vi "capex gui.vi"() -> ()   [LabVIEW 2013]
panel:
  in  "On quit":bool
  out "Heartbeat":bool
  in  "Tab Control":T1(tab)
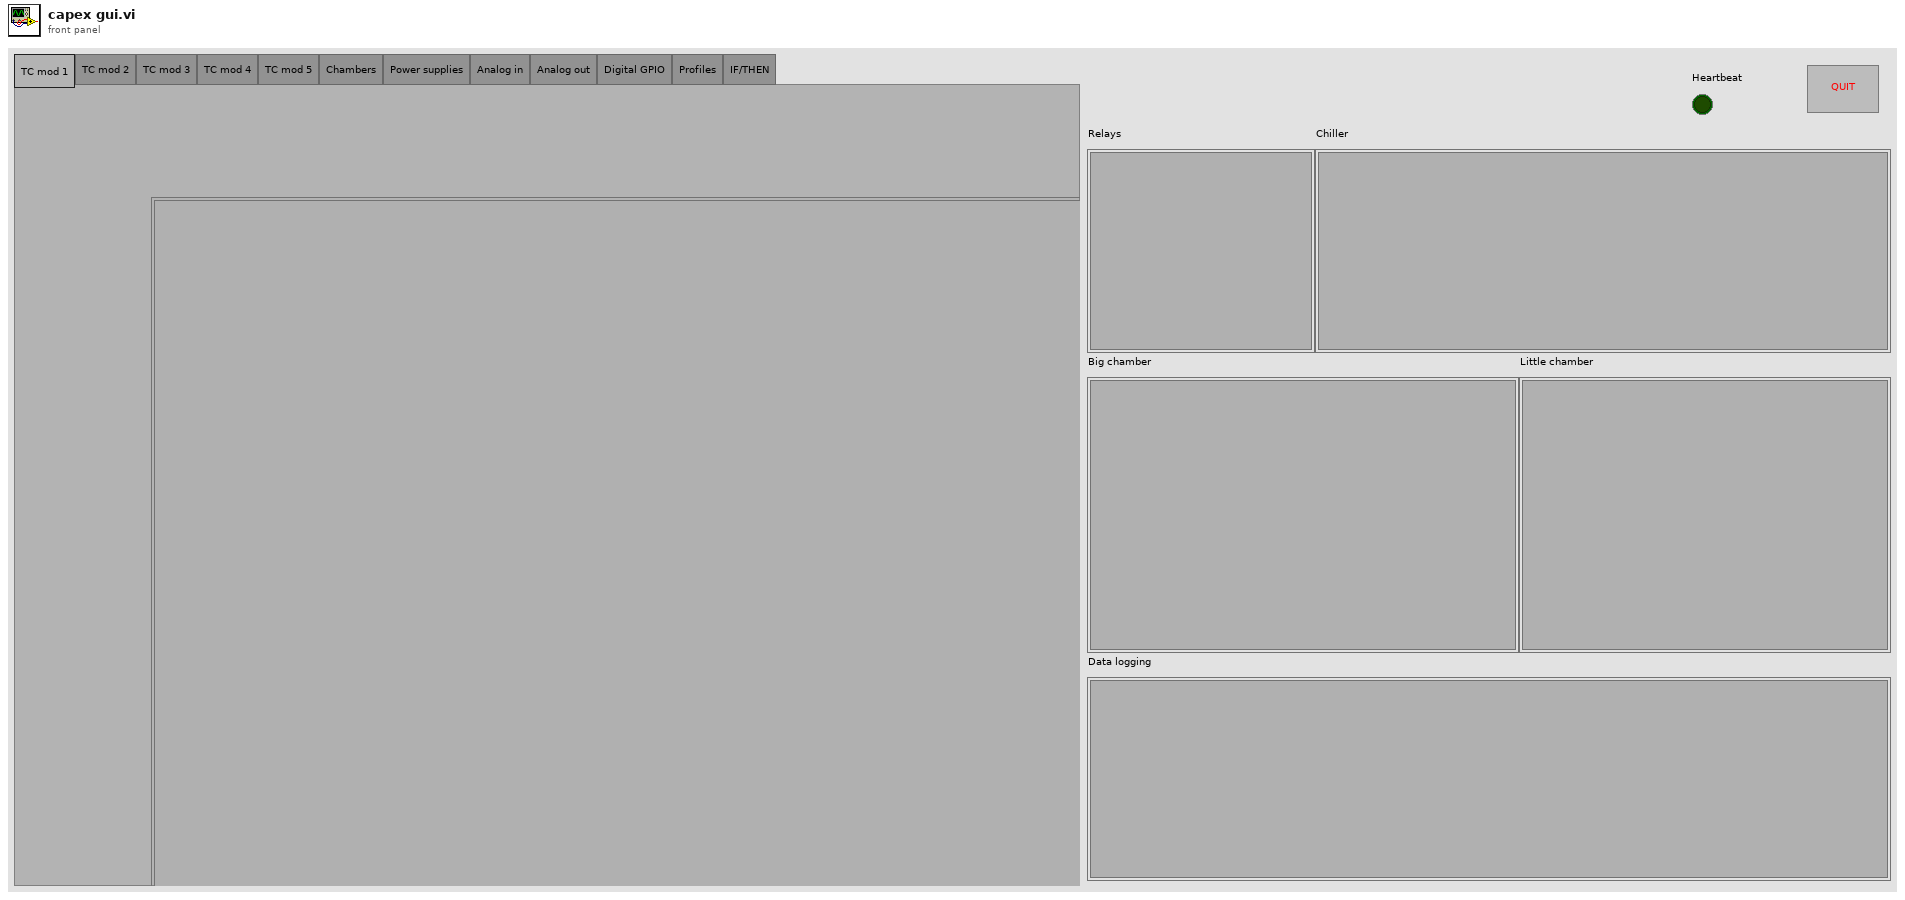
[diagram p1: front panel]
types:
  T1 = enum32{"TC mod 1", "TC mod 2", "TC mod 3", "TC mod 4", "TC mod 5", "Chambers", "Power supplies", "Analog in", "Analog out", "Digital GPIO", "Profiles", "IF/THEN"}
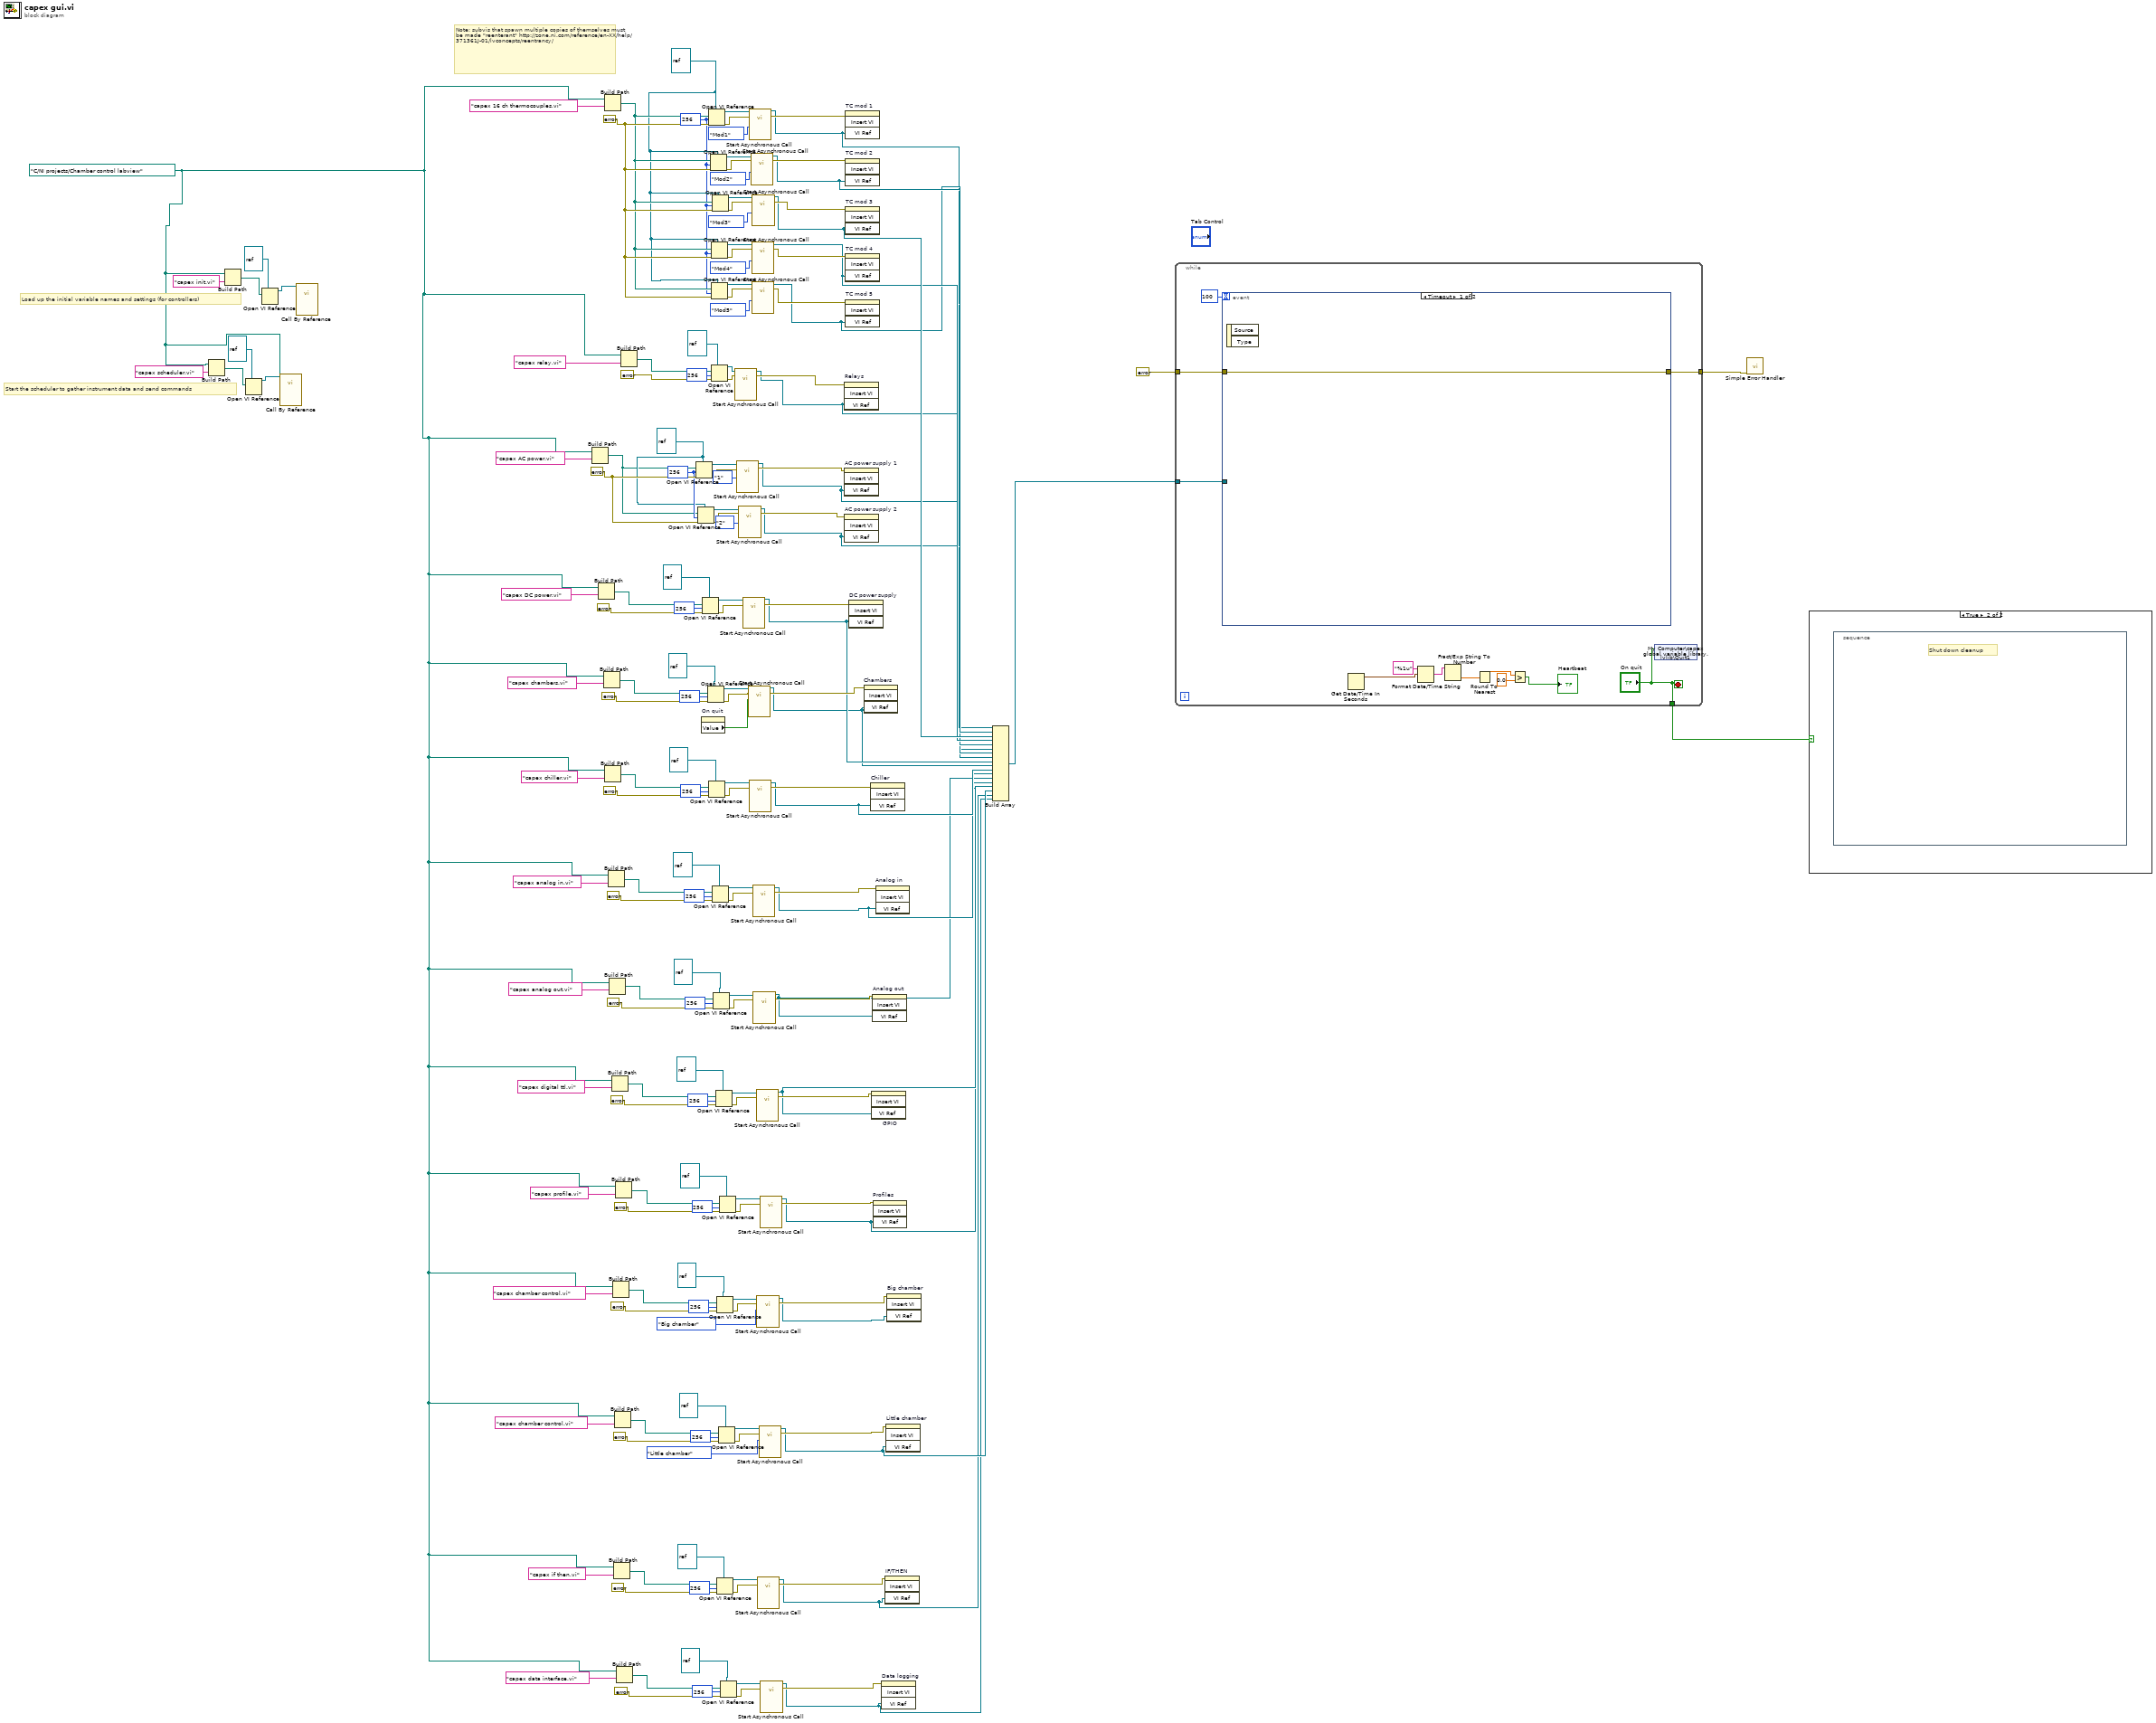
[diagram p0: block diagram]
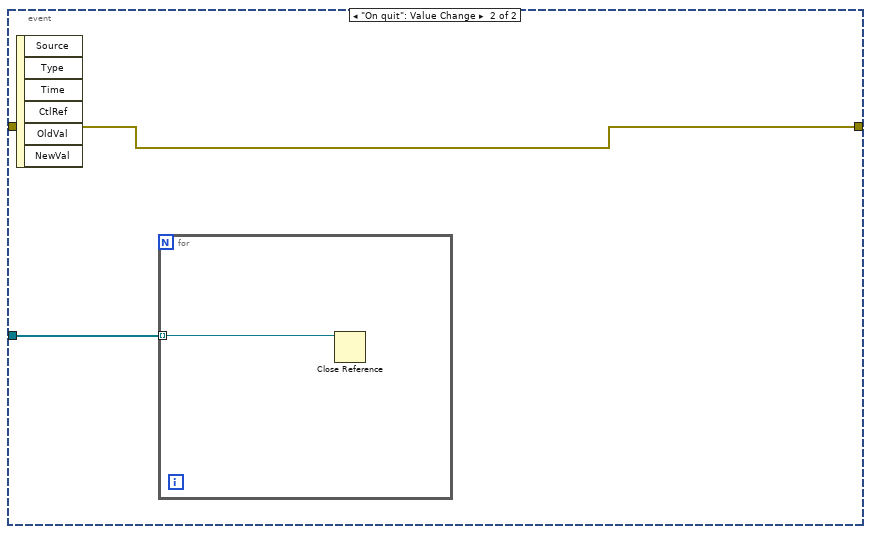
[diagram p3: hidden frame]
diagram:
  w138 = 256 ("options")
  w135 = refnum<vi> refnum ("type specifier VI Refnum (for type only)")
  w141 = errorcluster {"status"=FALSE, "code"=0, "source"=""} ("error out")
  w147 = 256 ("options")
  w148 = refnum<vi> refnum ("type specifier VI Refnum (for type only)")
  w162 = errorcluster {"status"=FALSE, "code"=0, "source"=""} ("error out")
  w11 = path "C:/NI projects/Chamber control labview"
  # "Start the scheduler to gather instrument data and send commands"
  # "Load up the initial variable names and settings (for controllers)"
  # "Note: subvis that spawn multiple copies of themselves must be made \"reenterant\" http://zone.ni.com/reference/en-XX/help/371361J-01/lvconcepts/reentrancy/"
  n1 = Build Path(base path=w11, name or relative path="capex scheduler.vi") -> (appended path=w5:path)
  n2 = Build Path(base path=w11, name or relative path="capex init.vi") -> (appended path=w9:path)
  n3 = Open VI Reference(type specifier VI Refnum (for type only)=refnum<vi> refnum, vi path=w5) -> (vi reference=w3:refnum<vi>)  [unwired: 4 in, 1 out]
  n4 = Open VI Reference(type specifier VI Refnum (for type only)=refnum<vi> refnum, vi path=w9) -> (vi reference=w7:refnum<vi>)  [unwired: 4 in, 1 out]
  n5 = call-by-ref "?"(reference=w3, "Path"=w11) -> ()  [unwired: 12 in, 2 out]
  n6 = call-by-ref "?"(reference=w7) -> ()  [unwired: 2 in, 11 out]
  n7 = Build Path(base path=w11, name or relative path="capex AC power.vi") -> (appended path=w134:path)
  n8 = Build Path(base path=w11, name or relative path="capex DC power.vi") -> (appended path=w119:path)
  n9 = Build Path(base path=w11, name or relative path="capex chambers.vi") -> (appended path=w111:path)
  n10 = Build Path(base path=w11, name or relative path="capex 16 ch thermocouples.vi") -> (appended path=w149:path)
  n11 = Build Path(base path=w11, name or relative path="capex chiller.vi") -> (appended path=w104:path)
  n12 = Build Path(base path=w11, name or relative path="capex analog in.vi") -> (appended path=w97:path)
  n13 = Build Path(base path=w11, name or relative path="capex analog out.vi") -> (appended path=w90:path)
  n14 = Build Path(base path=w11, name or relative path="capex digital ttl.vi") -> (appended path=w83:path)
  n15 = Build Path(base path=w11, name or relative path="capex chamber control.vi") -> (appended path=w44:path)
  n16 = Build Path(base path=w11, name or relative path="capex if then.vi") -> (appended path=w63:path)
  n17 = Build Path(base path=w11, name or relative path="capex chamber control.vi") -> (appended path=w37:path)
  n18 = Build Path(base path=w11, name or relative path="capex profile.vi") -> (appended path=w76:path)
  n19 = Build Path(base path=w11, name or relative path="capex data interface.vi") -> (appended path=w56:path)
  n20 = Build Path(base path=w11, name or relative path="capex relay.vi") -> (appended path=w168:path)
  n21 = Open VI Reference(type specifier VI Refnum (for type only)=w135, vi path=w134, options=w138, error in (no error)=w141) -> (vi reference=w143:refnum<vi>, error out=w142:errorcluster)  [unwired: 2 in]
  n22 = Open VI Reference(type specifier VI Refnum (for type only)=w135, vi path=w134, options=w138, error in (no error)=w141) -> (vi reference=w140:refnum<vi>, error out=w139:errorcluster)  [unwired: 2 in]
  n23 = property on="On quit" class="Bool (strict)"() -> ("Value"=w51:bool)  [unwired: 2 in, 2 out]
  n24 = Open VI Reference(type specifier VI Refnum (for type only)=refnum<vi> refnum, vi path=w119, options=256, error in (no error)=errorcluster {"status"=FALSE, "code"=0, "source"=""} ("error out")) -> (vi reference=w124:refnum<vi>, error out=w123:errorcluster)  [unwired: 2 in]
  n25 = Open VI Reference(type specifier VI Refnum (for type only)=refnum<vi> refnum, vi path=w111, options=256, error in (no error)=errorcluster {"status"=FALSE, "code"=0, "source"=""} ("error out")) -> (vi reference=w116:refnum<vi>, error out=w115:errorcluster)  [unwired: 2 in]
  n26 = Open VI Reference(type specifier VI Refnum (for type only)=w148, vi path=w149, options=w147, error in (no error)=w162) -> (vi reference=w165:refnum<vi>, error out=w164:errorcluster)  [unwired: 2 in]
  n27 = Open VI Reference(type specifier VI Refnum (for type only)=refnum<vi> refnum, vi path=w104, options=256, error in (no error)=errorcluster {"status"=FALSE, "code"=0, "source"=""} ("error out")) -> (vi reference=w109:refnum<vi>, error out=w108:errorcluster)  [unwired: 2 in]
  n28 = Open VI Reference(type specifier VI Refnum (for type only)=w148, vi path=w149, options=w147, error in (no error)=w162) -> (vi reference=w161:refnum<vi>, error out=w154:errorcluster)  [unwired: 2 in]
  n29 = Open VI Reference(type specifier VI Refnum (for type only)=w148, vi path=w149, options=w147, error in (no error)=w162) -> (vi reference=w159:refnum<vi>, error out=w156:errorcluster)  [unwired: 2 in]
  n30 = Open VI Reference(type specifier VI Refnum (for type only)=w148, vi path=w149, options=w147, error in (no error)=w162) -> (vi reference=w158:refnum<vi>, error out=w157:errorcluster)  [unwired: 2 in]
  n31 = Open VI Reference(type specifier VI Refnum (for type only)=refnum<vi> refnum, vi path=w168, options=256, error in (no error)=errorcluster {"status"=FALSE, "code"=0, "source"=""} ("error out")) -> (vi reference=w14:refnum<vi>, error out=w15:errorcluster)  [unwired: 2 in]
  n32 = Open VI Reference(type specifier VI Refnum (for type only)=w148, vi path=w149, options=w147, error in (no error)=w162) -> (vi reference=w160:refnum<vi>, error out=w155:errorcluster)  [unwired: 2 in]
  n33 = Open VI Reference(type specifier VI Refnum (for type only)=refnum<vi> refnum, vi path=w97, options=256, error in (no error)=errorcluster {"status"=FALSE, "code"=0, "source"=""} ("error out")) -> (vi reference=w102:refnum<vi>, error out=w101:errorcluster)  [unwired: 2 in]
  n34 = Open VI Reference(type specifier VI Refnum (for type only)=refnum<vi> refnum, vi path=w90, options=256, error in (no error)=errorcluster {"status"=FALSE, "code"=0, "source"=""} ("error out")) -> (vi reference=w95:refnum<vi>, error out=w94:errorcluster)  [unwired: 2 in]
  n35 = Open VI Reference(type specifier VI Refnum (for type only)=refnum<vi> refnum, vi path=w83, options=256, error in (no error)=errorcluster {"status"=FALSE, "code"=0, "source"=""} ("error out")) -> (vi reference=w88:refnum<vi>, error out=w87:errorcluster)  [unwired: 2 in]
  n36 = Open VI Reference(type specifier VI Refnum (for type only)=refnum<vi> refnum, vi path=w44, options=256, error in (no error)=errorcluster {"status"=FALSE, "code"=0, "source"=""} ("error out")) -> (vi reference=w49:refnum<vi>, error out=w48:errorcluster)  [unwired: 2 in]
  n37 = Open VI Reference(type specifier VI Refnum (for type only)=refnum<vi> refnum, vi path=w63, options=256, error in (no error)=errorcluster {"status"=FALSE, "code"=0, "source"=""} ("error out")) -> (vi reference=w68:refnum<vi>, error out=w67:errorcluster)  [unwired: 2 in]
  n38 = Open VI Reference(type specifier VI Refnum (for type only)=refnum<vi> refnum, vi path=w37, options=256, error in (no error)=errorcluster {"status"=FALSE, "code"=0, "source"=""} ("error out")) -> (vi reference=w42:refnum<vi>, error out=w41:errorcluster)  [unwired: 2 in]
  n39 = Open VI Reference(type specifier VI Refnum (for type only)=refnum<vi> refnum, vi path=w76, options=256, error in (no error)=errorcluster {"status"=FALSE, "code"=0, "source"=""} ("error out")) -> (vi reference=w81:refnum<vi>, error out=w80:errorcluster)  [unwired: 2 in]
  n40 = Open VI Reference(type specifier VI Refnum (for type only)=refnum<vi> refnum, vi path=w56, options=256, error in (no error)=errorcluster {"status"=FALSE, "code"=0, "source"=""} ("error out")) -> (vi reference=w61:refnum<vi>, error out=w60:errorcluster)  [unwired: 2 in]
  n41 = call-by-ref "Start Asynchronous Call"(reference=w14, error in=w15) -> (reference out=w12:refnum<vi>, error out=w13:errorcluster)  [unwired: 4 in]
  n42 = call-by-ref "Start Asynchronous Call"(reference=w143, error in=w142, "Enum"=enum16{"2", "1"}."1") -> (reference out=w128:refnum<vi>, error out=w137:errorcluster)  [unwired: 3 in]
  n43 = call-by-ref "Start Asynchronous Call"(reference=w140, error in=w139, "Enum"=enum16{"2", "1"}."2") -> (reference out=w127:refnum<vi>, error out=w136:errorcluster)  [unwired: 3 in]
  n44 = call-by-ref "Start Asynchronous Call"(reference=w124, error in=w123) -> (reference out=w31:refnum<vi>, error out=w118:errorcluster)  [unwired: 4 in]
  n45 = call-by-ref "Start Asynchronous Call"(reference=w116, error in=w115, "stop"=w51) -> (reference out=w30:refnum<vi>, error out=w75:errorcluster)  [unwired: 11 in]
  n46 = call-by-ref "Start Asynchronous Call"(reference=w165, error in=w164, "Enum"=enum16{"Mod1", "Mod2", "Mod3", "Mod4", "Mod5"}."Mod1") -> (reference out=w53:refnum<vi>, error out=w163:errorcluster)  [unwired: 11 in]
  n47 = call-by-ref "Start Asynchronous Call"(reference=w109, error in=w108) -> (reference out=w29:refnum<vi>, error out=w74:errorcluster)  [unwired: 1 in]
  n48 = call-by-ref "Start Asynchronous Call"(reference=w161, error in=w154, "Enum"=enum16{"Mod1", "Mod2", "Mod3", "Mod4", "Mod5"}."Mod2") -> (reference out=w132:refnum<vi>, error out=w153:errorcluster)  [unwired: 11 in]
  n49 = call-by-ref "Start Asynchronous Call"(reference=w159, error in=w156, "Enum"=enum16{"Mod1", "Mod2", "Mod3", "Mod4", "Mod5"}."Mod4") -> (reference out=w130:refnum<vi>, error out=w151:errorcluster)  [unwired: 11 in]
  n50 = call-by-ref "Start Asynchronous Call"(reference=w158, error in=w157, "Enum"=enum16{"Mod1", "Mod2", "Mod3", "Mod4", "Mod5"}."Mod5") -> (reference out=w129:refnum<vi>, error out=w150:errorcluster)  [unwired: 11 in]
  n51 = call-by-ref "Start Asynchronous Call"(reference=w160, error in=w155, "Enum"=enum16{"Mod1", "Mod2", "Mod3", "Mod4", "Mod5"}."Mod3") -> (reference out=w131:refnum<vi>, error out=w152:errorcluster)  [unwired: 11 in]
  n52 = call-by-ref "Start Asynchronous Call"(reference=w102, error in=w101) -> (reference out=w28:refnum<vi>, error out=w73:errorcluster)  [unwired: 1 in]
  n53 = call-by-ref "Start Asynchronous Call"(reference=w95, error in=w94) -> (reference out=w27:refnum<vi>, error out=w72:errorcluster)  [unwired: 4 in]
  n54 = call-by-ref "Start Asynchronous Call"(reference=w88, error in=w87) -> (reference out=w26:refnum<vi>, error out=w71:errorcluster)  [unwired: 1 in]
  n55 = call-by-ref "Start Asynchronous Call"(reference=w49, error in=w48, "Which chamber"=enum16{"Little chamber", "Big chamber"}."Big chamber") -> (reference out=w35:refnum<vi>, error out=w36:errorcluster)  [unwired: 11 in]
  n56 = call-by-ref "Start Asynchronous Call"(reference=w68, error in=w67) -> (reference out=w23:refnum<vi>, error out=w55:errorcluster)  [unwired: 12 in]
  n57 = call-by-ref "Start Asynchronous Call"(reference=w42, error in=w41, "Which chamber"=enum16{"Little chamber", "Big chamber"}."Little chamber") -> (reference out=w24:refnum<vi>, error out=w34:errorcluster)  [unwired: 11 in]
  n58 = call-by-ref "Start Asynchronous Call"(reference=w81, error in=w80) -> (reference out=w25:refnum<vi>, error out=w70:errorcluster)  [unwired: 12 in]
  n59 = call-by-ref "Start Asynchronous Call"(reference=w61, error in=w60) -> (reference out=w22:refnum<vi>, error out=w54:errorcluster)  [unwired: 12 in]
  n60 = invoke on="Relays" class="SubPanel" method="Insert VI"(error in=w13, "VI Ref"=w12) -> ()  [unwired: 2 in, 4 out]
  n61 = invoke on="AC power supply 1" class="SubPnl" method="Insert VI"(error in=w137, "VI Ref"=w128) -> ()  [unwired: 2 in, 4 out]
  n62 = invoke on="AC power supply 2" class="SubPanel" method="Insert VI"(error in=w136, "VI Ref"=w127) -> ()  [unwired: 2 in, 4 out]
  n63 = invoke on="TC mod 1" class="SubPanel" method="Insert VI"(error in=w163, "VI Ref"=w53) -> ()  [unwired: 2 in, 4 out]
  n64 = invoke on="TC mod 2" class="SubPnl" method="Insert VI"(error in=w153, "VI Ref"=w132) -> ()  [unwired: 2 in, 4 out]
  n65 = invoke on="TC mod 3" class="SubPnl" method="Insert VI"(error in=w152, "VI Ref"=w131) -> ()  [unwired: 2 in, 4 out]
  n66 = invoke on="TC mod 4" class="SubPnl" method="Insert VI"(error in=w151, "VI Ref"=w130) -> ()  [unwired: 2 in, 4 out]
  n67 = invoke on="TC mod 5" class="SubPnl" method="Insert VI"(error in=w150, "VI Ref"=w129) -> ()  [unwired: 2 in, 4 out]
  n68 = invoke on="DC power supply" class="SubPanel" method="Insert VI"(error in=w118, "VI Ref"=w31) -> ()  [unwired: 2 in, 4 out]
  n69 = invoke on="Chambers" class="SubPnl" method="Insert VI"(error in=w75, "VI Ref"=w30) -> ()  [unwired: 2 in, 4 out]
  n70 = invoke on="Chiller" class="SubPnl" method="Insert VI"(error in=w74, "VI Ref"=w29) -> ()  [unwired: 2 in, 4 out]
  n71 = invoke on="GPIO" class="SubPnl" method="Insert VI"(error in=w71, "VI Ref"=w26) -> ()  [unwired: 2 in, 4 out]
  n72 = invoke on="Analog out" class="SubPnl" method="Insert VI"(error in=w72, "VI Ref"=w27) -> ()  [unwired: 2 in, 4 out]
  n73 = invoke on="Profiles" class="SubPnl" method="Insert VI"(error in=w70, "VI Ref"=w25) -> ()  [unwired: 2 in, 4 out]
  n74 = invoke on="Analog in" class="SubPnl" method="Insert VI"(error in=w73, "VI Ref"=w28) -> ()  [unwired: 2 in, 4 out]
  n75 = invoke on="Data logging" class="SubPnl" method="Insert VI"(error in=w54, "VI Ref"=w22) -> ()  [unwired: 2 in, 4 out]
  n76 = invoke on="IF/THEN" class="SubPnl" method="Insert VI"(error in=w55, "VI Ref"=w23) -> ()  [unwired: 2 in, 4 out]
  n77 = invoke on="Little chamber" class="SubPnl" method="Insert VI"(error in=w34, "VI Ref"=w24) -> ()  [unwired: 2 in, 4 out]
  n78 = invoke on="Big chamber" class="SubPnl" method="Insert VI"(error in=w36, "VI Ref"=w35) -> ()  [unwired: 2 in, 4 out]
  n79 = Build Array(w53, w132, w131, w130, w129, w12, w128, w127, w31, w30, w29, w28, w27, w26, w25, w24, w23, w22) -> (w126:refnum<vi>[])
  n80 = while {
    tunnel: errorcluster {"status"=FALSE, "code"=0, "source"=""} ("error out") -> [w181]
    tunnel: [w180] -> w169
    tunnel: w126 -> [w176]
    tunnel: ["On quit"] -> w52
    stop <- "On quit" stop-if-true
    n81 = event shown="[0] Timeout" {
      selector: _ -> [_ _]
      dyn-events: _ -> [_ _]
      timeout: 100 -> [_ _]
      tunnel: w181 -> [w182 w184]
      tunnel: [w182 w184] -> w180
      tunnel: w176 -> [_ w183]
      event Timeout {
        n82 = event-data() -> ()  [unwired: 1 in, 2 out]
      }
      event "On quit": Value Change {
        n83 = event-data() -> ()  [unwired: 1 in, 6 out]
        n84 = for {
          tunnel: w183 -> [w185] mode=indexing
          n85 = Close Reference(reference=w185) -> ()  [unwired: 1 in, 1 out]
        }
      }
    }
    n86 = Get Date/Time In Seconds() -> (seconds since 1Jan1904=w174:timestamp)
    n87 = Format Date/Time String(time format string (%c)="%1u", seconds (now)=w174) -> (date/time string=w171:string)  [unwired: 1 in]
    n88 = Fract/Exp String To Number(string=w171) -> (number=w172:dbl)  [unwired: 3 in, 1 out]
    n89 = Round To Nearest(number=w172) -> (nearest integer value=w175:dbl)
    n90 = Greater?(x=w175, y=0.0) -> (0:→"Heartbeat":bool)
    n91 = shared-variable "My Computer\\capex global variable library.lvlib\\Quit1"("On quit") -> ()  [unwired: 1 in, 1 out]
  }
  n92 = call <vilib>:"Simple Error Handler.vi"("error in (no error)"=w169) -> ()  [unwired: 4 in, 5 out]
  n93 = case shown="True" w52 {
    frame False {
    }
    frame True {
      n94 = stacked-sequence {
        frame #0 {
          # "Shut down cleanup"
        }
      }
    }
  }
